vi "Set Date.vi"(8 "error in (no error)":errorcluster, 10 "Selected Date":timestamp, 11 "Budgetizer in":refnum<class "Budgetizer.lvclass">) -> (0 "error out":errorcluster, 3 "Budgetizer out":refnum<class "Budgetizer.lvclass">)   [LabVIEW 2018, in "Budgetizer.lvclass"]
uses:
  Budgetizer.lvclass
  Budgetizer.lvclass/Budgetizer.ctl
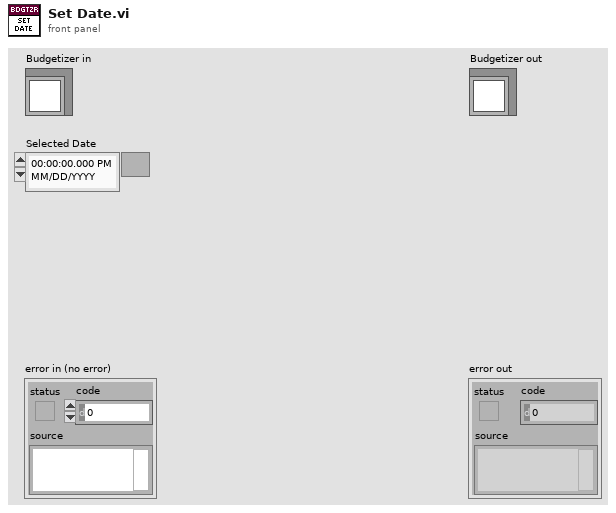
[diagram p1: front panel]
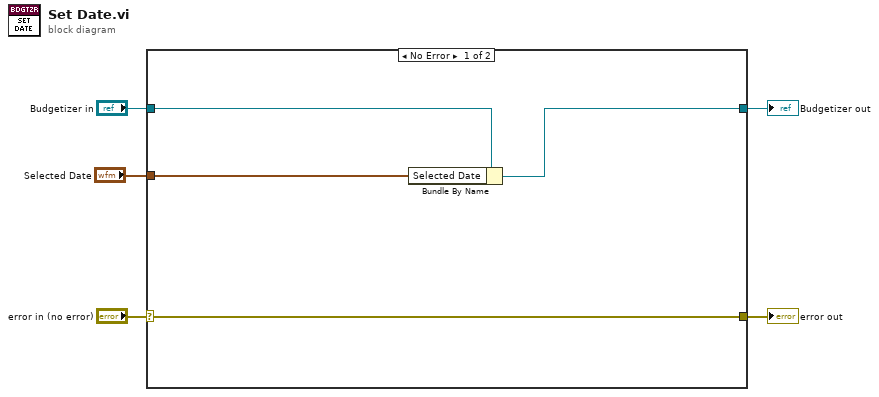
[diagram p0: block diagram]
diagram:
  n1 = case shown="No Error" "error in (no error)" {
    selector: "error in (no error)" -> [w9 w11]
    tunnel: [w9 w11] -> w4
    tunnel: [w7 w10] -> w2
    tunnel: "Budgetizer in" -> [w8 w10]
    tunnel: "Selected Date" -> [w6 _]
    frame No Error {
      n2 = Bundle By Name(cluster=w8, "Selected Date"=w6) -> (w7:refnum<class "Budgetizer.lvclass">)
    }
    frame Error {
    }
  }
  "error out" <- w4
  "Budgetizer out" <- w2
